vi "test single REQ.vi"() -> ()   [LabVIEW 2018, in "LV-0mq-Julia_roundtrip-lib.lvlib"]
uses:
  LV-0mq-Julia_roundtrip-lib.lvlib
  Commands.ctl
  <vilib>/addons/zeromq/zmq_socket.lvclass
panel:
  out "short err code":u8
  out "roundtrip time":dbl
  out "detailed err description":string
  out "JSON data":string
  out "binary data":u8[](array[numeric])
  out "server response":string
  in  "data to send":string="hello"
  out "error out":errorcluster
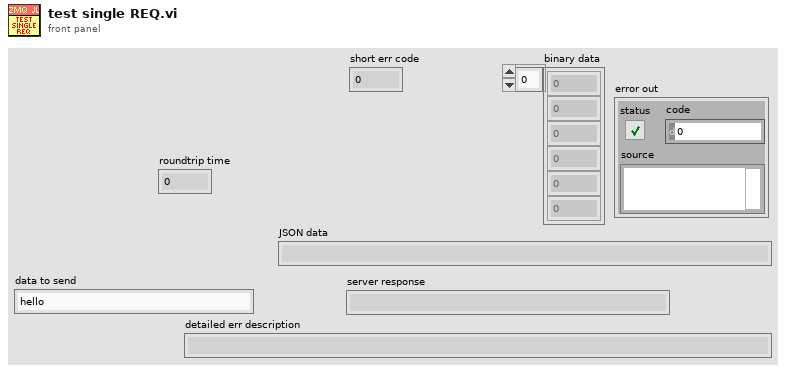
[diagram p1: front panel]
types:
  T1 = typedef "LV-0mq-Julia_roundtrip-lib.lvlib/Commands.ctl" = enum16{"Start Jl-server & Init LV-client", "Send request & Get response ", "Stop Jl-server & Cleanup LV-client", "Cleanup LV-client", "Start Jl-server", "Stop Jl-server", "Init LV-Client", "Cleanup LV-Client", "(not allowed)", "Set LV Client state", "Set Jl Server state", "set ZMQ timeout", "read ZMQ timeout", "read-out state"}
  T2 = typedef "LV-0mq-Julia_roundtrip-lib.lvlib/detailed error info.ctl" = cluster{"exception_or_info":string, "trace":T3[]}
  T3 = typedef "LV-0mq-Julia_roundtrip-lib.lvlib/StackFrame.ctl" = cluster{"frame_summary":string, "func":string, "linfo":string, "file":string, "line":i32, "pointer":u64, "from_c":bool, "inlined":bool}
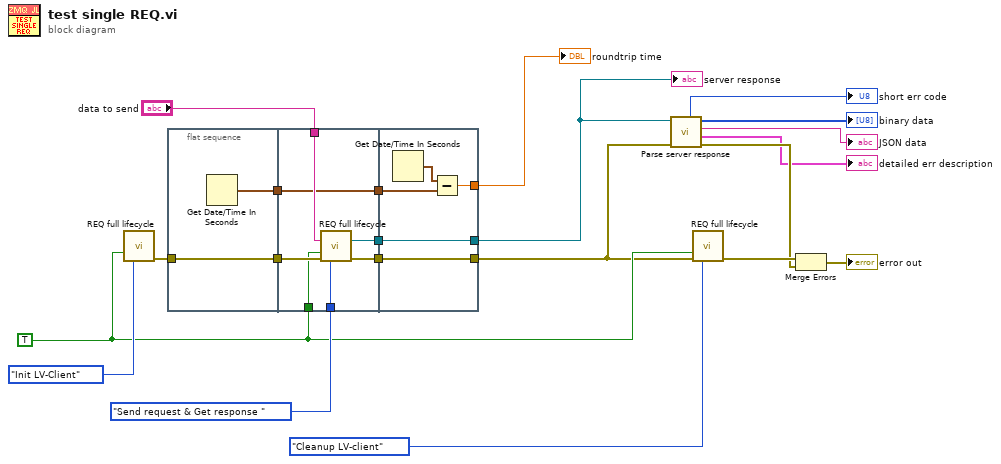
[diagram p0: block diagram]
diagram:
  w16 = TRUE ("Force command")
  n1 = call "REQ full lifecycle.vi"("Force command"=w16, "command"=Commands."Init LV-Client") -> ("error out"=w20:errorcluster)  [unwired: 7 in, 6 out]
  n2 = flat-sequence {
    tunnel: w20 -> [w23]
    tunnel: [w23] -> w5
    tunnel: [w22] -> w4
    tunnel: Commands."Send request & Get response " ("command") -> [w29]
    tunnel: w16 -> [w28]
    tunnel: "data to send" -> [w27]
    tunnel: [w26] -> w7
    tunnel: [w25] -> w6
    tunnel: w5 -> [w30]
    tunnel: w4 -> [w24]
    tunnel: [w24] -> w3
    tunnel: [w34] -> w13
    tunnel: [w35] -> w14
    tunnel: w7 -> [w35]
    tunnel: w6 -> [w34]
    tunnel: w3 -> [w32]
    tunnel: [w31] -> w2
    frame #0 {
      n3 = Get Date/Time In Seconds() -> (seconds since 1Jan1904=w22:timestamp)
    }
    frame #1 {
      n4 = call "REQ full lifecycle.vi"("data to send"=w27, "Force command"=w28, "error in"=w30, "command"=w29) -> ("socket out"=w26:refnum<class "zmq_socket.lvclass">, "error out"=w25:errorcluster)  [unwired: 5 in, 5 out]
    }
    frame #2 {
      n5 = Get Date/Time In Seconds() -> (seconds since 1Jan1904=w33:timestamp)
      n6 = Subtract(x=w33, y=w32) -> (x-y=w31:dbl)
    }
  }
  n7 = call "Parse server response.vi"("error in (no error)"=w13, "server response in"=w14) -> ("error out"=w11:errorcluster, "detailed error info"=→"detailed err description":T2, "JSON out"=→"JSON data":string, "binary data"=→"binary data":u8[], "return code"=→"short err code":u8)  [unwired: 2 in, 3 out]
  n8 = call "REQ full lifecycle.vi"("Force command"=w16, "error in"=w13, "command"=Commands."Cleanup LV-client") -> ("error out"=w18:errorcluster)  [unwired: 6 in, 6 out]
  n9 = Merge Errors(w18, w11) -> (→"error out":errorcluster)
  "server response" <- w14
  "roundtrip time" <- w2
